vi "ADRESS LIST.vi"() -> ()   [LabVIEW 2025]
panel:
  out "error out":errorcluster
  out "listener address list":i16[](array[numeric])
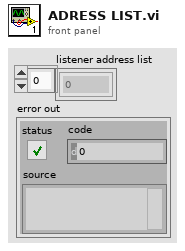
[diagram p1: front panel]
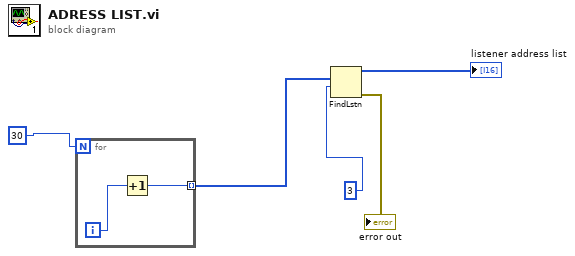
[diagram p0: block diagram]
diagram:
  n1 = for {
    N: 30 -> [_]
    tunnel: [w6] -> w4 mode=indexing
    i -> [w7]
    n2 = Increment(x=w7) -> (x+1=w6:i32)
  }
  n3 = FindLstn(5:3, 6:w4) -> (0:→"error out":errorcluster, 3:→"listener address list":i16[])  [unwired: 2 in, 2 out]
